vi "DoorNeedingSpellParamsStack.vi"(8 "error in (no error)":errorcluster, 10 "room2":refnum<class "Room.lvclass">, 11 "room1":refnum<class "Room.lvclass">) -> (0 "error out":errorcluster, 2 "HierarchyParams":variant[](array[variant]), 3 "DoorNeedingSpell":refnum<class "DoorNeedingSpell.lvclass">)   [LabVIEW 2020, in "DoorNeedingSpell.lvclass"]
uses:
  DoorNeedingSpell.lvclass
  E:/GitHub/Design-Patterns-GoF_-_NI-LV/Creational/GoFcommonClasses/ConcreteMazeSite/Door/Door.lvclass
  Room/Room.lvclass
  Door/Protected/property/Read DoorParams.vi
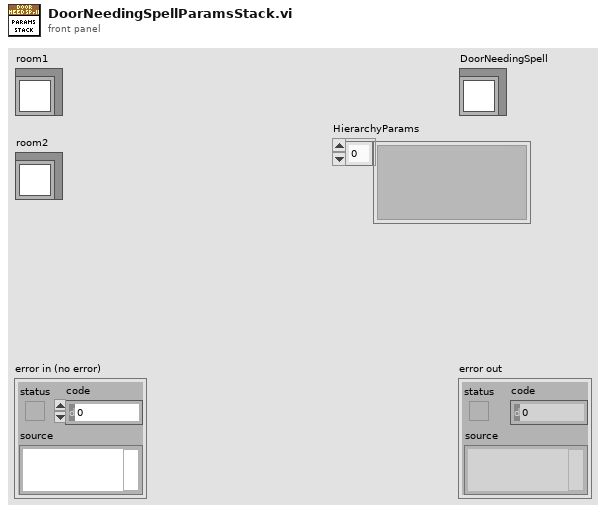
[diagram p1: front panel]
types:
  T1 = typedef "Door.lvclass/DoorParams.ctl" = cluster{"room1":refnum<class "Room.lvclass">, "room2":refnum<class "Room.lvclass">}
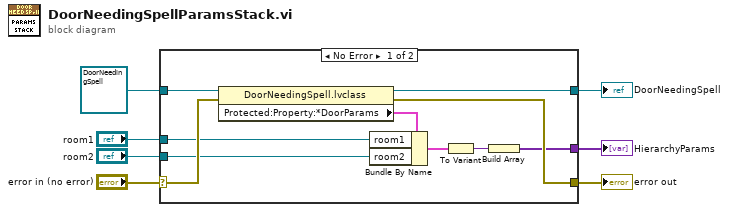
[diagram p0: block diagram]
diagram:
  n1 = case shown="No Error" "error in (no error)" {
    selector: "error in (no error)" -> [w10 w19]
    tunnel: [w15 w19] -> w6
    tunnel: refnum<class "DoorNeedingSpell.lvclass"> refnum ("Milk") -> [w17 w18]
    tunnel: [w16 w18] -> w4
    tunnel: [w14 _] -> w3
    tunnel: "room1" -> [w9 _]
    tunnel: "room2" -> [w8 _]
    frame No Error {
      n2 = property class="DoorNeedingSpell.lvclass"(reference=w17, error in=w10) -> (reference out=w16:refnum<class "DoorNeedingSpell.lvclass">, error out=w15:errorcluster, "Protected:Property:*DoorParams"=w11:T1)
      n3 = Bundle By Name(cluster=w11, "room1"=w9, "room2"=w8) -> (w13:T1)
      n4 = To Variant(anything=w13) -> (Variant=w12:variant)
      n5 = Build Array(w12) -> (w14:variant[])
    }
    frame Error {
    }
  }
  "error out" <- w6
  "DoorNeedingSpell" <- w4
  "HierarchyParams" <- w3
